vi "ImageControlProbe.vi"(1 "Image In":T1) -> (0 "Breakpoint":bool)   [LabVIEW 2018]
uses:
  <vilib>/vision/Image Controls.llb/IMAQ Image.ctl
panel:
  out "Image":T1(plugin-control)
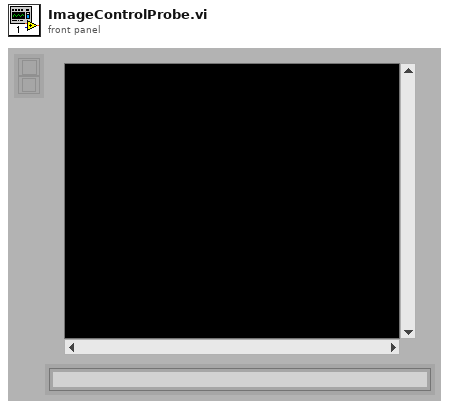
[diagram p1: front panel]
types:
  T1 = typedef "IMAQ Image.ctl" = refnum<image>
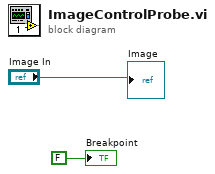
[diagram p0: block diagram]
diagram:
  "Breakpoint" <- FALSE ("Breakpoint")
  "Image" <- "Image In"
